vi "rethinkdb_msg_unhandled.vi"(8 "error in (no error)":errorcluster, 11 "message":string) -> (0 "error out":errorcluster)   [LabVIEW 2017]
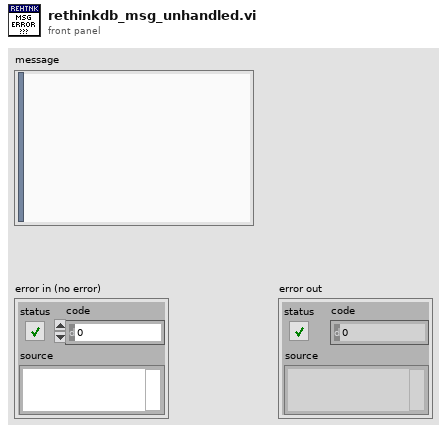
[diagram p1: front panel]
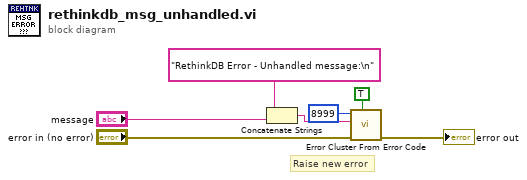
[diagram p0: block diagram]
diagram:
  # "Raise new error"
  n1 = Concatenate Strings("RethinkDB Error - Unhandled message:\n" ("error message (\"\")"), "message") -> (w1:string)
  n2 = call <vilib>:"Error Cluster From Error Code.vi"("show call chain? (False)"=TRUE, "error in (no error)"="error in (no error)", "error message (\"\")"=w1, "error code (0)"=8999) -> ("error out"=→"error out":errorcluster)  [unwired: 5 in]
